vi "Action Engine Auto Reset Test.vi"() -> ()   [LabVIEW 2021]
uses:
  Controls/Timer Actions.ctl
panel:
  in  "Time Duration (s)":dbl=2.0
  out "Clock Output":bool
  out "Time Elapsed":dbl
  in  "Stop Button":bool
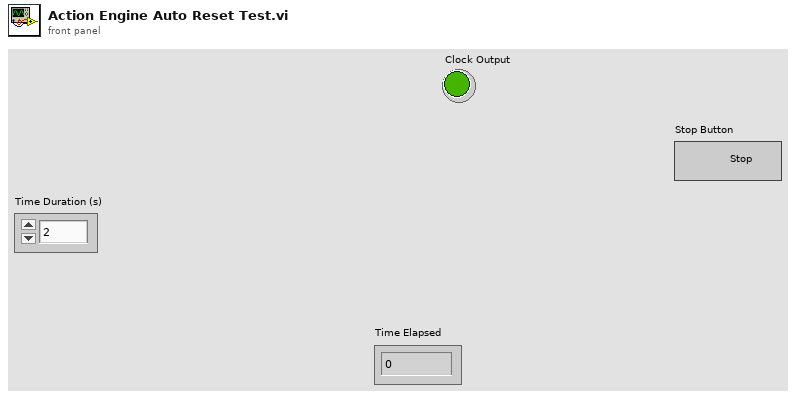
[diagram p1: front panel]
types:
  T1 = typedef "Timer Actions.ctl" = enum16{"Start Timer", "Restart Timer", "Check Timer", "Pause Timer", "Reset Timer", "Exit Timer"}
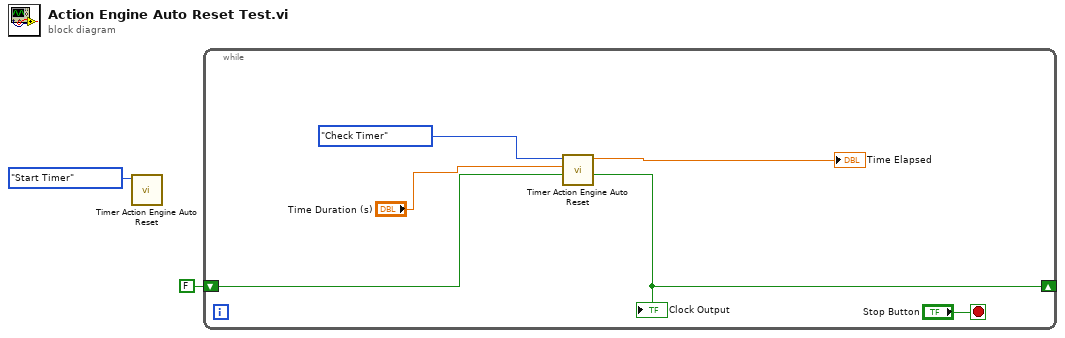
[diagram p0: block diagram]
diagram:
  n1 = call "Timer Action Engine Auto Reset.vi"("Action"=Timer_Actions."Start Timer") -> ()  [unwired: 7 in, 4 out]
  n2 = while {
    shift-right: [w5] -> _
    shift-left: FALSE ("Clock Output") -> [w4]
    stop <- "Stop Button" stop-if-true
    n3 = call "Timer Action Engine Auto Reset.vi"("Current State"=w4, "Time Duration (s)"="Time Duration (s)", "Action"=Timer_Actions."Check Timer") -> ("Clock Output"=w5:bool, "Time Elapsed"=→"Time Elapsed":dbl)  [unwired: 5 in, 2 out]
    "Clock Output" <- w5
  }
